vi "determine warnings case structure.vi"() -> ()   [LabVIEW 2014]
panel:
  out "warning?":bool
  out "warning text":string
  in  "min temp":dbl
  in  "max temp":dbl
  in  "current temp.":dbl
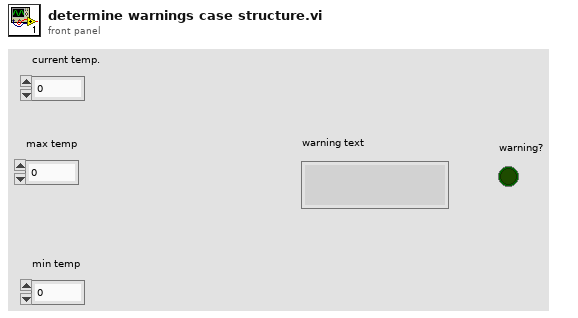
[diagram p1: front panel]
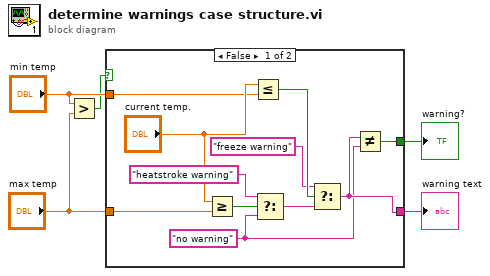
[diagram p0: block diagram]
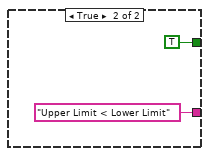
[diagram p2: hidden frame]
diagram:
  n1 = Greater?(x="min temp", y="max temp") -> (0:w1:bool)
  n2 = case shown="False" w1 {
    tunnel: [w10 "Upper Limit < Lower Limit"] -> w5
    tunnel: [w8 TRUE ("warning?")] -> w4
    tunnel: "min temp" -> [w7 _]
    tunnel: "max temp" -> [w6 _]
    frame False {
      w9 = "no warning"
      n3 = Greater Or Equal?(x="current temp.", y=w6) -> (x >= y?=w14:bool)
      n4 = Less Or Equal?(x="current temp.", y=w7) -> (x <= y?=w15:bool)
      n5 = Select(t="heatstroke warning", s=w14, f=w9) -> (s? t:f=w11:string)
      n6 = Select(t="freeze warning", s=w15, f=w11) -> (s? t:f=w10:string)
      n7 = Not Equal?(x=w10, y=w9) -> (x != y?=w8:bool)
    }
    frame True {
    }
  }
  "warning text" <- w5
  "warning?" <- w4
